vi "בדיקת זמן מיתוג הממסר 4.vi"(7 "resultUserPrompt":bool, 8 "error":errorcluster, 11 "Path for Log":path) -> (0 "error out":errorcluster, 1 "בטוח כן/לא":bool, 2 "בדיקת זמן מיתוג הממסר":dbl)   [LabVIEW 2015]
uses:
  <instrlib>/niDMM/nidmm.llb/niDMM Function.ctl
  <instrlib>/niDMM/nidmm.llb/niDMM Resolution in Digits.ctl
  <vilib>/DAQmx/write.llb/DAQmx Write (Digital Bool 1Line 1Point).vi
  <vilib>/DAQmx/create/channels.llb/DAQmx Create Channel (DO-Digital Output).vi
  <instrlib>/niDMM/nidmm.llb/niDMM Configure Measurement Digits.vi
  <vilib>/DAQmx/miscellaneous.llb/DAQmx Fill In Error Info.vi
panel:
  in  "התחל":bool
  # "Right-Click to\nexplain error"
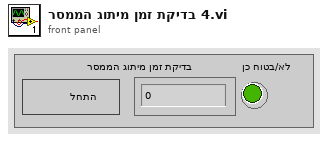
[diagram p1: front panel]
types:
  T1 = enum32{"Invalid", "Standard", "Closed", "Hidden", "Minimized", "Maximized"}
  T2 = typedef "niDMM Function.ctl" = enum16{"DC Volts", "AC Volts", "DC Current", "AC Current", "2-wire Resistance", "4-wire Resistance", "Diode", "Frequency", "Period", "AC Volts DC Coupled", "Capacitance", "Inductance", "Temperature"}
  T3 = typedef "niDMM Resolution in Digits.ctl" = dbl
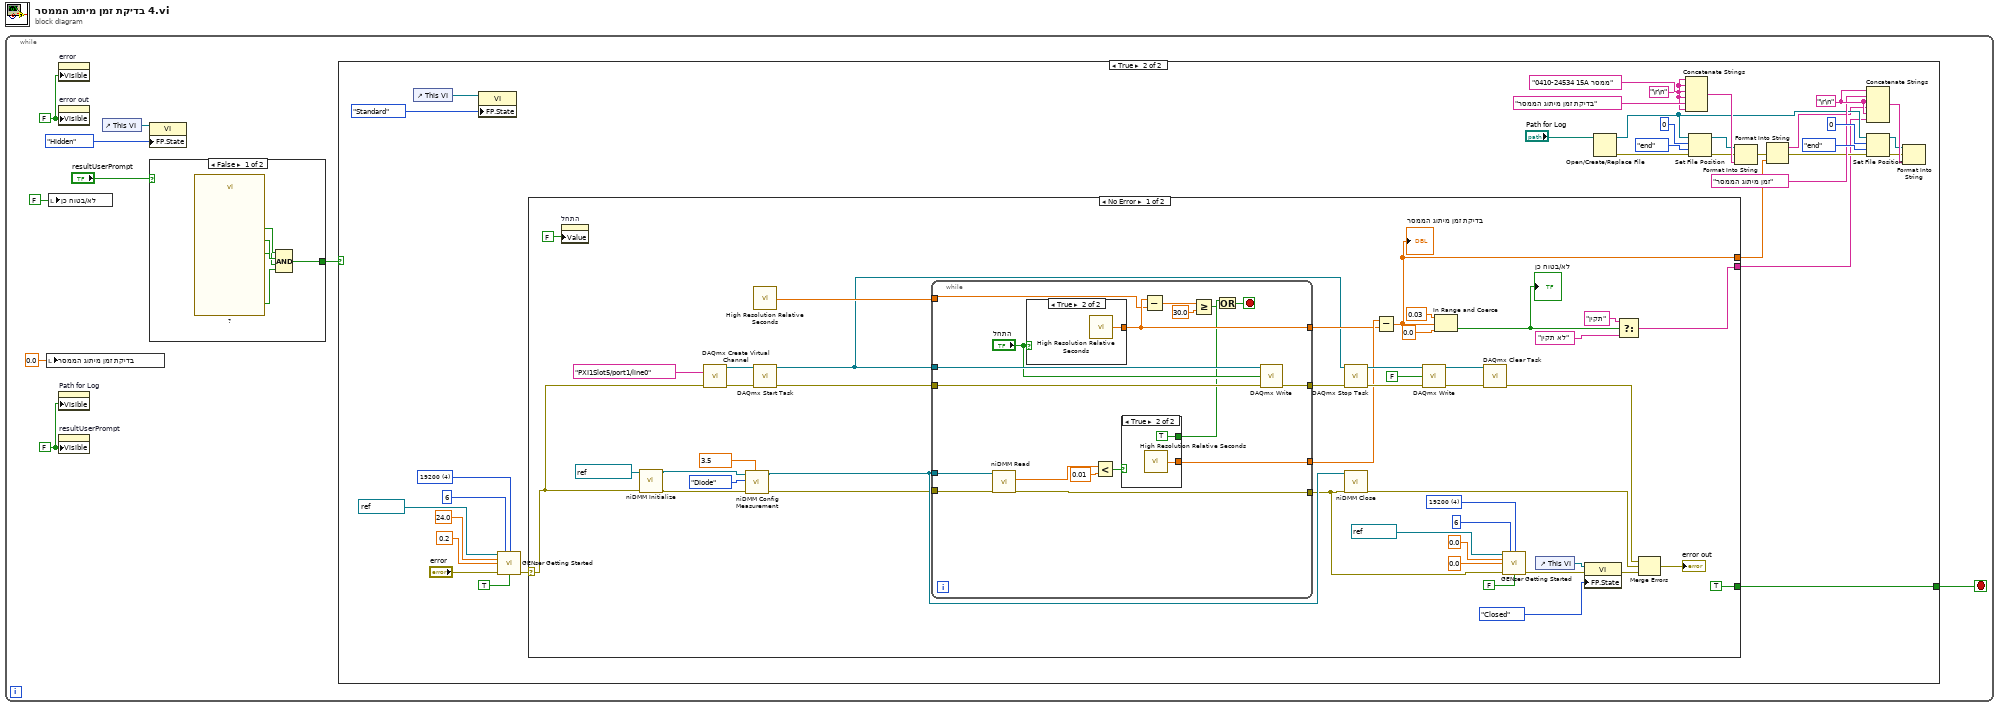
[diagram p0: block diagram]
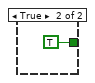
[diagram p2: hidden frame]
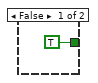
[diagram p3: hidden frame]
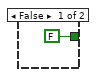
[diagram p4: hidden frame]
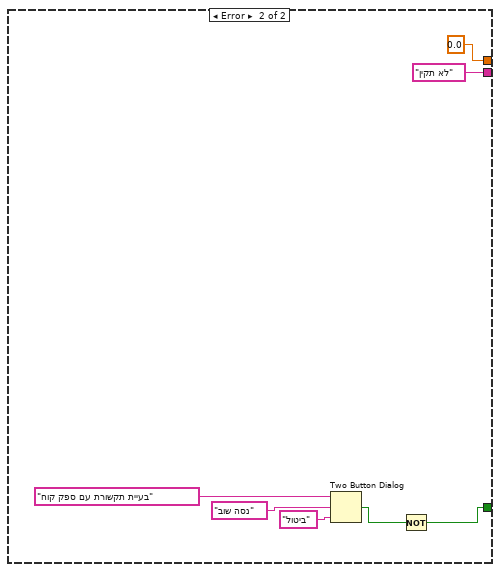
[diagram p6: hidden frame]
diagram:
  n1 = while {
    stop <- w1 stop-if-true
    w2 = FALSE ("Visible")
    w9 = FALSE ("Visible")
    n2 = local write "בדיקת זמן מיתוג הממסר"(0.0 ("בדיקת זמן מיתוג הממסר")) -> ()
    n3 = local write "בטוח כן/לא"(FALSE ("בטוח כן/לא")) -> ()
    n4 = property on="error" class="Clust (strict)"("Visible"=w9) -> ()  [unwired: 2 in, 2 out]
    n5 = property on="error out" class="Clust (strict)"("Visible"=w9) -> ()  [unwired: 2 in, 2 out]
    n6 = property on="Path for Log" class="Path"("Visible"=w2) -> ()  [unwired: 2 in, 2 out]
    n7 = property on="resultUserPrompt" class="Bool (strict)"("Visible"=w2) -> ()  [unwired: 2 in, 2 out]
    n8 = control-ref of="This VI"() -> (w8:refnum<vi>)
    n9 = property class="VI"(reference=w8, "FP.State"=T1."Hidden" ("Front Panel Window:State")) -> ()  [unwired: 1 in, 2 out]
    n10 = case shown="False" "resultUserPrompt" {
      tunnel: [w10 TRUE] -> w6
      frame False {
        n11 = call "?"() -> ("הדקי הרב מודד"=w11:bool, "(מגע שלילי (מעטפת"=w12:bool, "A מגע חיובי"=w13:bool, "OK"=w14:bool)  [unwired: 15 in, 1 out]
        n12 = Compound Arithmetic op=AND(w14, w13, w12, w11) -> (w10:bool)
      }
      frame True {
      }
    }
    n13 = case shown="True" w6 {
      tunnel: [TRUE ("T button?") w43] -> w1
      frame False {
      }
      frame True {
        w26 = "\r\n"
        w33 = "\r\n"
        w46 = u16 4 items=["1200", "2400", "4800", "9600", "19200"] ("BAUD")
        n14 = control-ref of="This VI"() -> (w42:refnum<vi>)
        n15 = property class="VI"(reference=w42, "FP.State"=T1."Standard" ("Front Panel Window:State")) -> ()  [unwired: 1 in, 2 out]
        n16 = call "GENser Getting Started.vi"("VISA"=refnum<visa-resource-name> "COM6", "GEN Addr"=i16 6, "BAUD"=w46, "Voltage Limit"=24.0, "Current Limit"=0.2, "error"="error", "Output On (T)"=TRUE) -> ("error out"=w48:errorcluster)  [unwired: 5 in, 3 out]
        n17 = case shown="No Error" w48 {
          selector: w48 -> [w57 _]
          tunnel: [TRUE ("T button?") w118] -> w43
          tunnel: [w71 0.0] -> w18
          tunnel: [w67 "לא תקין"] -> w17
          frame No Error {
            w60 = T3 3.5 items=["3 1/2"=3.5, "4 1/2"=4.5, "5 1/2"=5.5, "6 1/2"=6.5, "7 1/2"=7.5] ("Resolution in Digits")
            w89 = u16 4 items=["1200", "2400", "4800", "9600", "19200"] ("BAUD")
            n18 = property on="התחל" class="Bool (strict)"("Value"=FALSE ("data")) -> ()  [unwired: 2 in, 2 out]
            n19 = call <instrlib>:"niDMM Initialize.vi"("error in (no error)"=w57, "Instrument Descriptor"=refnum<k15> "PXI1Slot9") -> ("error out"=w58:errorcluster, "instrument handle out"=w59:refnum<k15>)  [unwired: 8 in]
            n20 = call-poly <vilib>:"DAQmx Create Virtual Channel.vi"("lines"=tag "PXI1Slot5/port1/line0", "error in"=w57) -> ("task out"=w64:refnum<k21>, "error out"=w65:errorcluster)  [unwired: 12 in]
            n21 = call-poly <instrlib>:"niDMM Config Measurement.vi"("Resolution in Digits"=w60, "error in (no error)"=w58, "Function"=niDMM_Function."Diode", "instrument handle"=w59) -> ("error out"=w54:errorcluster, "instrument handle out"=w56:refnum<k15>)  [unwired: 6 in]
            n22 = call <vilib>:"High Resolution Relative Seconds.vi"() -> ("relative seconds"=w62:dbl)
            n23 = call <vilib>:"DAQmx Start Task.vi"("task/channels in"=w64, "error in"=w65) -> ("task out"=w55:refnum<k21>, "error out"=w53:errorcluster)  [unwired: 12 in]
            n24 = while {
              tunnel: [w107] -> w78
              tunnel: [w113] -> w79
              tunnel: w55 -> [w112]
              tunnel: w53 -> [w111]
              tunnel: w62 -> [w106]
              tunnel: w56 -> [w99]
              tunnel: w54 -> [w98]
              tunnel: [w97] -> w52
              tunnel: [w96] -> w51
              stop <- w103 stop-if-true
              n25 = call <instrlib>:"niDMM Read.vi"("error in (no error)"=w98, "instrument handle"=w99) -> ("error out"=w96:errorcluster, "Measurement"=w110:dbl)  [unwired: 7 in, 1 out]
              n26 = case shown="True" "התחל" {
                tunnel: [_ w117] -> w107
                frame False {
                }
                frame True {
                  n27 = call <vilib>:"High Resolution Relative Seconds.vi"() -> ("relative seconds"=w117:dbl)
                }
              }
              n28 = Less?(x=w110, y=0.01) -> (x < y?=w100:bool)
              n29 = case shown="True" w100 {
                tunnel: [_ w116] -> w113
                tunnel: [FALSE TRUE] -> w102
                frame False {
                }
                frame True {
                  n30 = call <vilib>:"High Resolution Relative Seconds.vi"() -> ("relative seconds"=w116:dbl)
                }
              }
              n31 = Subtract(x=w107, y=w106) -> (x-y=w105:dbl)
              n32 = Greater Or Equal?(x=w105, y=30.0) -> (x >= y?=w101:bool)
              n33 = Or(x=w102, y=w101) -> (x .or. y?=w103:bool)
              n34 = call-poly <vilib>:"DAQmx Write.vi"("task/channels in"=w112, "data"="התחל", "error in"=w111) -> ("error out"=w97:errorcluster)  [unwired: 10 in, 2 out]
            }
            n35 = call <vilib>:"DAQmx Stop Task.vi"("task/channels in"=w55, "error in"=w52) -> ("task out"=w84:refnum<k21>, "error out"=w83:errorcluster)  [unwired: 12 in]
            n36 = call <instrlib>:"niDMM Close.vi"("error in (no error)"=w51, "instrument handle"=w56) -> ("error out"=w75:errorcluster)  [unwired: 9 in]
            n37 = Subtract(x=w79, y=w78) -> (x-y=w71:dbl)
            "בדיקת זמן מיתוג הממסר" <- w71
            n38 = call-poly <vilib>:"DAQmx Write.vi"("task/channels in"=w84, "data"=FALSE, "error in"=w83) -> ("task out"=w81:refnum<k21>, "error out"=w82:errorcluster)  [unwired: 10 in, 1 out]
            n39 = In Range and Coerce(upper limit=0.03, x=w71, lower limit=0.0) -> (In Range?=w68:bool)  [unwired: 1 out]
            "בטוח כן/לא" <- w68
            n40 = call <vilib>:"DAQmx Clear Task.vi"("task in"=w81, "error in"=w82) -> ("error out"=w76:errorcluster)  [unwired: 13 in]
            n41 = call "GENser Getting Started.vi"("VISA"=refnum<visa-resource-name> "COM6", "GEN Addr"=i16 6, "BAUD"=w89, "Voltage Limit"=0.0, "Current Limit"=0.0, "error"=w51, "Output On (T)"=FALSE) -> ("error out"=w88:errorcluster)  [unwired: 5 in, 3 out]
            n42 = control-ref of="This VI"() -> (w87:refnum<vi>)
            n43 = property class="VI"(reference=w87, error in=w88, "FP.State"=T1."Closed" ("Front Panel Window:State")) -> (error out=w74:errorcluster)  [unwired: 1 out]
            n44 = Select(t="תקין", s=w68, f="לא תקין") -> (s? t:f=w67:string)
            n45 = Merge Errors(w76, w75, w74) -> (→"error out":errorcluster)
          }
          frame Error {
            n46 = Two Button Dialog(message="בעיית תקשורת עם ספק קוח", 1:"ביטול" ("F button name (\"Cancel\")"), 2:"נסה שוב" ("T button name (\"OK\")")) -> (T button?=w119:bool)
            n47 = Not(x=w119) -> (.not. x?=w118:bool)
          }
        }
        n48 = Open/Create/Replace File(file path (use dialog)="Path for Log") -> (refnum out=w22:refnum<file>, error out=w23:errorcluster)  [unwired: 5 in, 1 out]
        n49 = Concatenate Strings(w33, w33, "0410-24534 15A ממסר", w33, "בדיקת זמן מיתוג הממסר", w33) -> (w37:string)
        n50 = Set File Position(offset (in bytes) (0)=i64 0, refnum=w22, from (0:start)=enum16{"start", "end", "current"}."end", error in=w23) -> (refnum out=w34:refnum<file>, error out=w32:errorcluster)
        n51 = Format Into String(initial string=w34, error in=w32, w37) -> (error out=w21:errorcluster)  [unwired: 1 in, 1 out]
        n52 = Format Into String(error in=w21, w18) -> (resulting string=w19:string, error out=w20:errorcluster)  [unwired: 2 in]
        n53 = Concatenate Strings(w26, "זמן מיתוג הממסר", w26, w19, w26, w17) -> (w31:string)
        n54 = Set File Position(offset (in bytes) (0)=i64 0, refnum=w22, from (0:start)=enum16{"start", "end", "current"}."end", error in=w20) -> (refnum out=w29:refnum<file>, error out=w30:errorcluster)
        n55 = Format Into String(initial string=w29, error in=w30, w31) -> ()  [unwired: 1 in, 2 out]
      }
    }
  }
